vi "read from xml.vi"(8 "error constant":errorcluster) -> (0 "error out":errorcluster, 3 "DAQ Config":T1)   [LabVIEW 2017]
uses:
  Control/Config chanel.ctl
  <vilib>/Utility/xml.llb/Read From XML File(string).vi
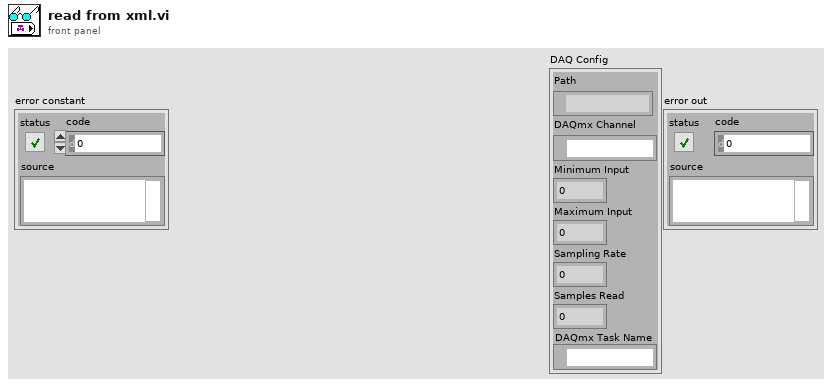
[diagram p1: front panel]
types:
  T1 = typedef "Config chanel.ctl" = cluster{"Path":path, "DAQmx Channel":tag, "Minimum Input":dbl, "Maximum Input":dbl, "Sampling Rate":dbl, "Samples Read":dbl, "DAQmx Task Name":refnum<k21>}
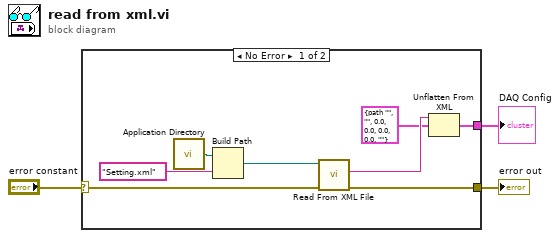
[diagram p0: block diagram]
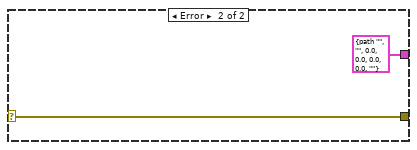
[diagram p2: hidden frame]
diagram:
  n1 = case shown="No Error" "error constant" {
    selector: "error constant" -> [w6 w13]
    tunnel: [w5 w13] -> w2
    tunnel: [w4 T1 {"Path"=path "", "DAQmx Channel"="", "Minimum Input"=0.0, "Maximum Input"=0.0, "Sampling Rate"=0.0, "Samples Read"=0.0, "DAQmx Task Name"=""} ("DAQ Config")] -> w1
    frame No Error {
      n2 = call <vilib>:"Application Directory.vi"() -> ("Application Directory"=w11:path)
      n3 = Build Path(base path=w11, name or relative path="Setting.xml") -> (appended path=w9:path)
      n4 = call-poly <vilib>:"Read From XML File.vi"("error in (no error)"=w6, "XML File Path"=w9) -> ("error out"=w5:errorcluster, "XML Elements"=w8:string)  [unwired: 7 in, 1 out]
      n5 = Unflatten From XML(xml string=w8, type=T1 {"Path"=path "", "DAQmx Channel"="", "Minimum Input"=0.0, "Maximum Input"=0.0, "Sampling Rate"=0.0, "Samples Read"=0.0, "DAQmx Task Name"=""} ("DAQ Config")) -> (value=w4:T1)  [unwired: 1 in, 1 out]
    }
    frame Error {
    }
  }
  "error out" <- w2
  "DAQ Config" <- w1
